vi "Problem 7.vi"() -> (2 "Prime Numbers":u32[](array[numeric]), 3 "10001st Prime":u32)   [LabVIEW 2013, in "Problem 7.lvlib"]
uses:
  Problem 7.lvlib
  Problem 3/Problem 3.lvlib
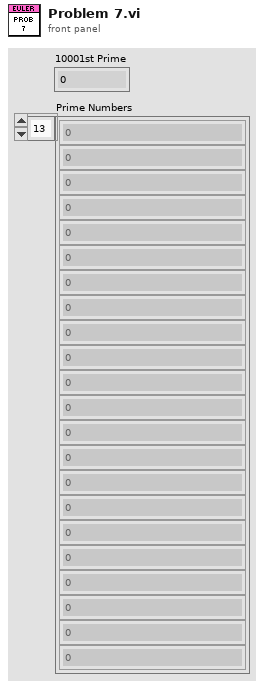
[diagram p1: front panel]
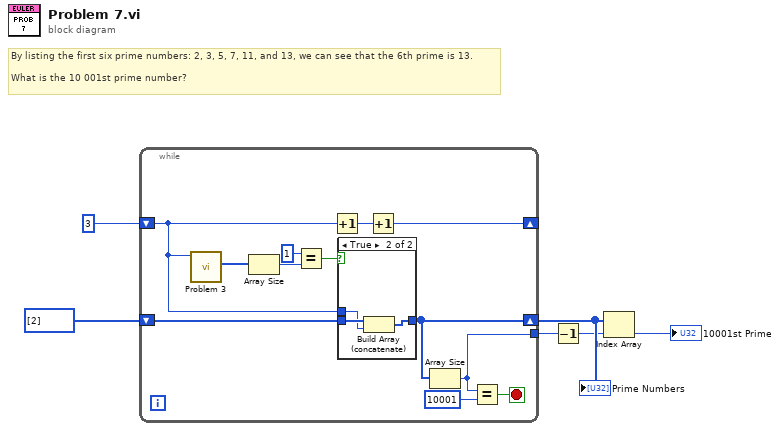
[diagram p0: block diagram]
diagram:
  # "By listing the first six prime numbers: 2, 3, 5, 7, 11, and 13, we can see that the 6th prime is 13.\n\nWhat is the 10 001st prime number?"
  n1 = while {
    shift-right: [w17] -> _
    shift-left: u32 3 -> [w12]
    shift-right: [w11] -> w4
    shift-left: u32[] [2] -> [w13]
    tunnel: [w8] -> w3
    stop <- w9 stop-if-true
    n2 = call "Problem 3.vi"("Number to Factor"=w12) -> ("List of Factors"=w16:u64[])  [unwired: 9 in, 1 out]
    n3 = Array Size(array=w16) -> (size(s)=w15:i32)
    n4 = Equal?(x=1, y=w15) -> (x = y?=w14:bool)
    n5 = Increment(x=w12) -> (x+1=w18:u32)
    n6 = case shown="True" w14 {
      tunnel: w13 -> [w19 w22]
      tunnel: w12 -> [_ w21]
      tunnel: [w19 w20] -> w11
      frame False {
      }
      frame True {
        n7 = Build Array (concatenate)(w22, w21) -> (w20:u32[])
      }
    }
    n8 = Increment(x=w18) -> (x+1=w17:u32)
    n9 = Array Size(array=w11) -> (size(s)=w8:i32)
    n10 = Equal?(x=w8, y=10001) -> (x = y?=w9:bool)
  }
  "Prime Numbers" <- w4
  n11 = Decrement(x=w3) -> (x-1=w2:i32)
  n12 = Index Array(array=w4, index=w2) -> (element=→"10001st Prime":u32)
